vi "Power Create Request.vi"(8 "error in (no error)":errorcluster, 11 "Simple Reason String":string) -> (0 "error out":errorcluster, 3 "Handle":i64)   [LabVIEW 2020, in "Power Requests.lvlib"]
uses:
  Power Requests.lvlib
  kernel32.dll
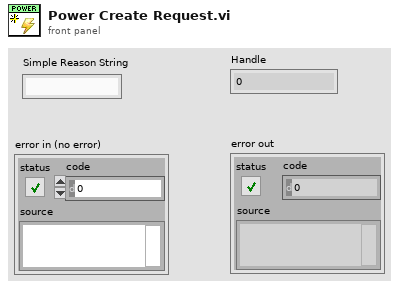
[diagram p1: front panel]
types:
  T1 = cluster{"Version":u32, "Flags":u32, "SimpleReasonString":u64}
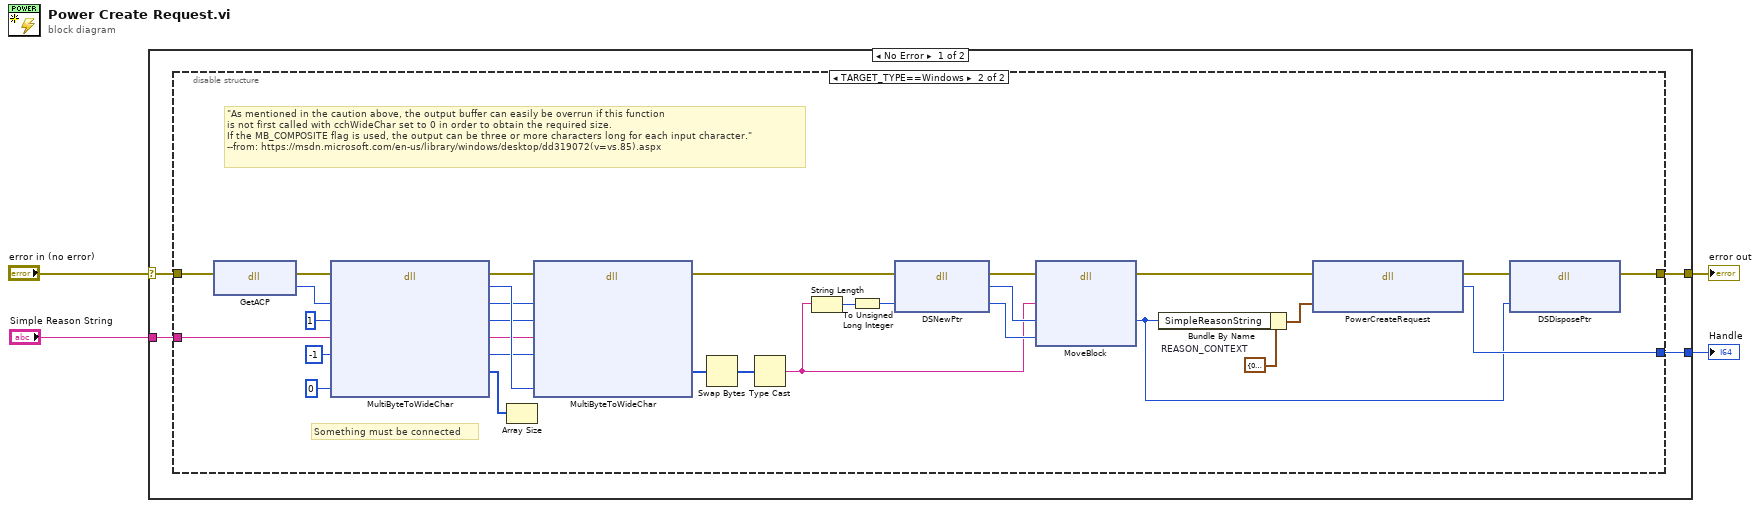
[diagram p0: block diagram]
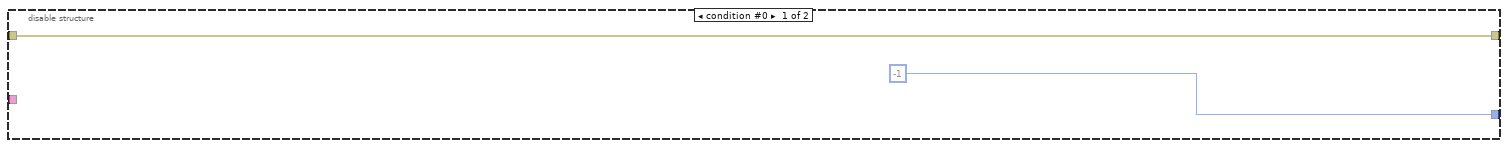
[diagram p2: hidden frame]
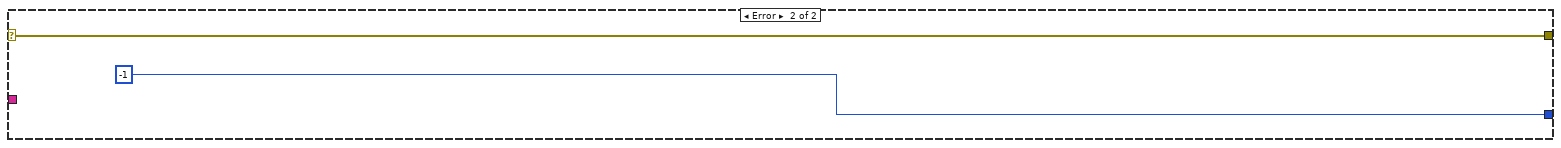
[diagram p3: hidden frame]
diagram:
  n1 = case shown="No Error" "error in (no error)" {
    selector: "error in (no error)" -> [w6 w42]
    tunnel: [w8 w42] -> w4
    tunnel: "Simple Reason String" -> [w5 _]
    tunnel: [w7 i64 -1] -> w1
    frame No Error {
      n2 = disable-structure shown="TARGET_TYPE==Windows" {
        disable-tunnel: [w10 w12] -> w8
        disable-tunnel: [i64 -1 w40] -> w7
        disable-tunnel: w6 -> [w10 w27]
        disable-tunnel: w5 -> [_ w26]
        frame condition #0 {
        }
        frame condition #1 (active) {
          w20 = T1 {"Version"=0, "Flags"=1, "SimpleReasonString"=0}  # REASON_CONTEXT
          # "\"As mentioned in the caution above, the output buffer can easily be overrun if this function\nis not first called with cchWideChar set to 0 in order to obtain the required size.\nIf the MB_COMPOSITE flag is used, the output can be three or more characters long for each input character.\"\n--from: https://msdn.microsoft.com/en-us/library/windows/desktop/dd319072(v=vs.85).aspx"
          # "Something must be connected"
          n3 = dll-call lib="kernel32.dll" fn="GetACP" ("GetACP()")(error in=w27) -> (error out=w32:errorcluster, "UINT"=w28:u32)  [unwired: 2 in, 1 out]
          n4 = dll-call lib="kernel32.dll" fn="MultiByteToWideChar"(error in=w32, "_In_ CodePage"=w28, "_In_ dwFlags"=u32 1 ("MB_PRECOMPOSED"), "_In_ lpMultByteStr"=w26, "_In_ cbMultByte"=-1 ("nChars"), "_In_ cchWideChar"=0 ("nWStr")) -> (error out=w33:errorcluster, "INT"=w38:i32, "_In_ CodePage"=w34:u32, "_In_ dwFlags"=w35:u32, "_In_ lpMultByteStr"=w36:string, "_In_ cbMultByte"=w37:i32, "_Out_opt_ lpWideCharStr"=w39:u16[])  [unwired: 4 in, 1 out]
          n5 = Array Size(array=w39) -> ()  [unwired: 1 out]
          n6 = dll-call lib="kernel32.dll" fn="MultiByteToWideChar"(error in=w33, "_In_ CodePage"=w34, "_In_ dwFlags"=w35, "_In_ lpMultByteStr"=w36, "_In_ cbMultByte"=w37, "_In_ cchWideChar"=w38) -> (error out=w22:errorcluster, "_Out_opt_ lpWideCharStr"=w18:u16[])  [unwired: 9 in, 1 out]
          n7 = Swap Bytes(anything=w18) -> (byte swapped=w15:u16[])
          n8 = Type Cast(x=w15) -> (*(type *) &x=w17:string)  [unwired: 1 in]
          n9 = String Length(string=w17) -> (length=w14:i32)
          n10 = To Unsigned Long Integer(number=w14) -> (unsigned 32bit integer=w16:u32)
          n11 = dll-call lib="LabVIEW" fn="DSNewPtr"(error in=w22, "size"=w16) -> (error out=w25:errorcluster, "return type"=w23:u64, "size"=w24:u32)  [unwired: 2 in, 1 out]
          n12 = dll-call lib="LabVIEW" fn="MoveBlock"(error in=w25, "pSrc"=w17, "pDst"=w23, "size"=w24) -> (error out=w21:errorcluster, "pDst"=w11:u64)  [unwired: 5 in, 1 out]
          n13 = Bundle By Name(cluster=w20, "SimpleReasonString"=w11) -> (w19:T1)
          n14 = dll-call lib="kernel32.dll" fn="PowerCreateRequest"(error in=w21, "_In_ PREASON_CONTEXT"=w19) -> (error out=w13:errorcluster, "HANDLE"=w40:i64)  [unwired: 3 in, 1 out]
          n15 = dll-call lib="LabVIEW" fn="DSDisposePtr"(error in=w13, "Pointer"=w11) -> (error out=w12:errorcluster)  [unwired: 4 in, 1 out]
        }
      }
    }
    frame Error {
    }
  }
  "error out" <- w4
  "Handle" <- w1
